vi "subprocess event queue pair.vi"(7 "bag action":T1, 9 "all in":refnum<user-event>[](array[refnum]), 11 "user event":refnum<user-event>) -> (1 "all out":refnum<user-event>[](array[refnum]))   [LabVIEW 2020]
uses:
  que event bag action.ctl
  server talkto message type.ctl
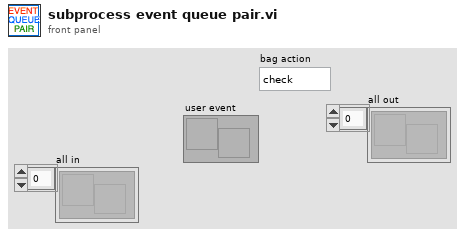
[diagram p1: front panel]
types:
  T1 = typedef "que event bag action.ctl" = enum16{"check", "add", "init"}
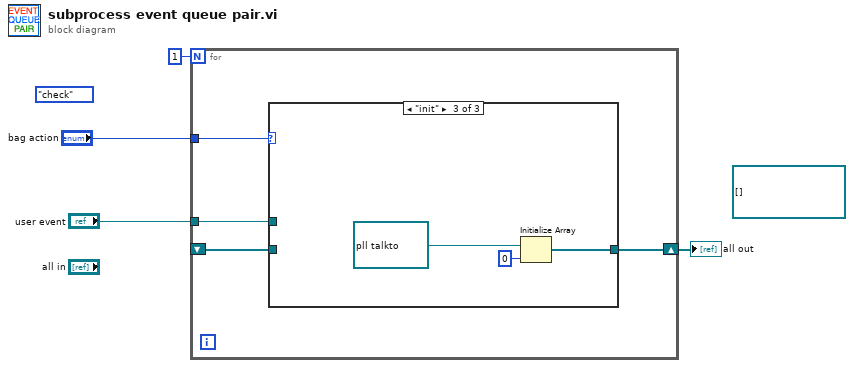
[diagram p0: block diagram]
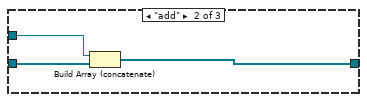
[diagram p3: hidden frame]
diagram:
  (unwired) refnum<user-event>[] [] ("all subprocesse")
  (unwired) que_event_bag_action."check" ("bag action")
  n1 = for {
    N: 1 -> [_]
    tunnel: "bag action" -> [w8]
    shift-right: [w7] -> w2
    shift-left: _ -> [w6]
    tunnel: "user event" -> [w5]
    n2 = case shown="\"init\"" w8 {
      tunnel: [w9 w10 w15] -> w7
      tunnel: w6 -> [w9 w12 _]
      tunnel: w5 -> [_ w11 _]
      frame "check", Default {
      }
      frame "add" {
        n3 = Build Array (concatenate)(w11, w12) -> (w10:refnum<user-event>[])
      }
      frame "init" {
        n4 = Initialize Array(refnum<user-event> refnum ("user event out"), 0 ("dimension size")) -> (w15:refnum<user-event>[])
      }
    }
  }
  "all out" <- w2
